vi "NET_Cube_HSV.vi"(8 "Read(F) Write(T)":bool, 9 "V In":dbl, 10 "S In":dbl, 11 "H In":dbl) -> (1 "V Out":dbl, 2 "S Out":dbl, 3 "H Out":dbl)   [LabVIEW 2017]
uses:
  <vilib>/Rock Robotics/Network Tables/NT Read Numeric Array.vi
  <vilib>/Rock Robotics/Network Tables/NT Write Numeric Array.vi
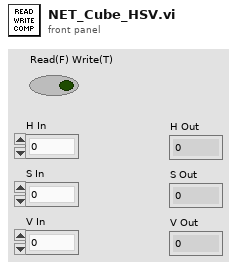
[diagram p1: front panel]
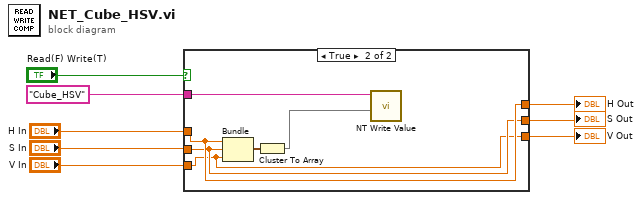
[diagram p0: block diagram]
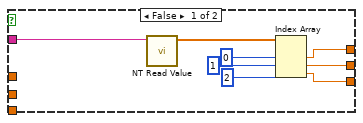
[diagram p2: hidden frame]
diagram:
  n1 = case shown="True" "Read(F) Write(T)" {
    tunnel: "Cube_HSV" ("Name") -> [w16 w22]
    tunnel: [w11 w18] -> w6
    tunnel: [w10 w19] -> w5
    tunnel: [w9 w17] -> w4
    tunnel: "H In" -> [_ w19]
    tunnel: "S In" -> [_ w18]
    tunnel: "V In" -> [_ w17]
    frame False {
      n2 = call-poly <vilib>:"NT Read Value.vi"("Name"=w16) -> ("Numeric Array"=w15:dbl[])  [unwired: 9 in, 1 out]
      n3 = Index Array(array=w15, index #1=0 ("index"), index #2=1 ("index"), index #3=2 ("index")) -> (element #1=w10:dbl, element #2=w11:dbl, element #3=w9:dbl)
    }
    frame True {
      n4 = Bundle("H In"=w19, "S In"=w18, "V In"=w17) -> (w21:cluster{"H In":dbl, "S In":dbl, "V In":dbl})  [unwired: 1 in]
      n5 = Cluster To Array(cluster=w21) -> (array=w20:dbl[])
      n6 = call-poly <vilib>:"NT Write Value.vi"("Numeric Array"=w20, "Name"=w22) -> ()  [unwired: 9 in, 1 out]
    }
  }
  "S Out" <- w6
  "V Out" <- w4
  "H Out" <- w5
